vi "main bascula.vi"() -> ()   [LabVIEW 2019]
uses:
  Controls/semafor.ctl
  Controls/Estats.ctl
panel:
  out "Semafor":T1
  out "pedestrian":bool
  in  "Boolean":bool
  in  "stop":bool
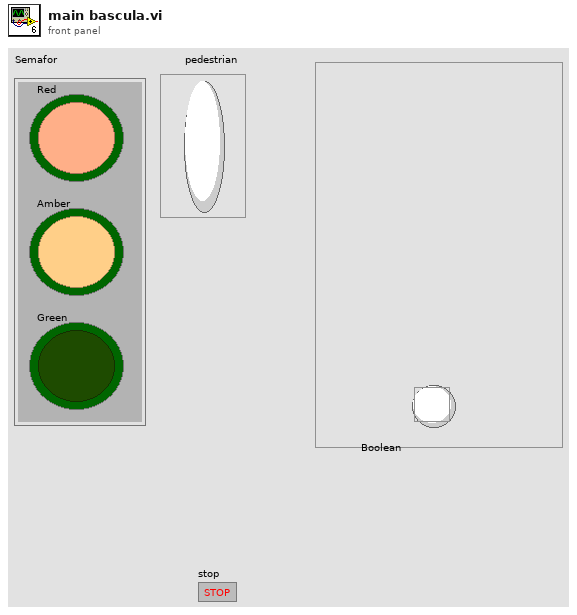
[diagram p1: front panel]
types:
  T1 = typedef "semafor.ctl" = cluster{"Red":bool, "Amber":bool, "Green":bool}
  T2 = typedef "Estats.ctl" = enum16{"Init", "Green", "Amber-red", "red", "amber"}
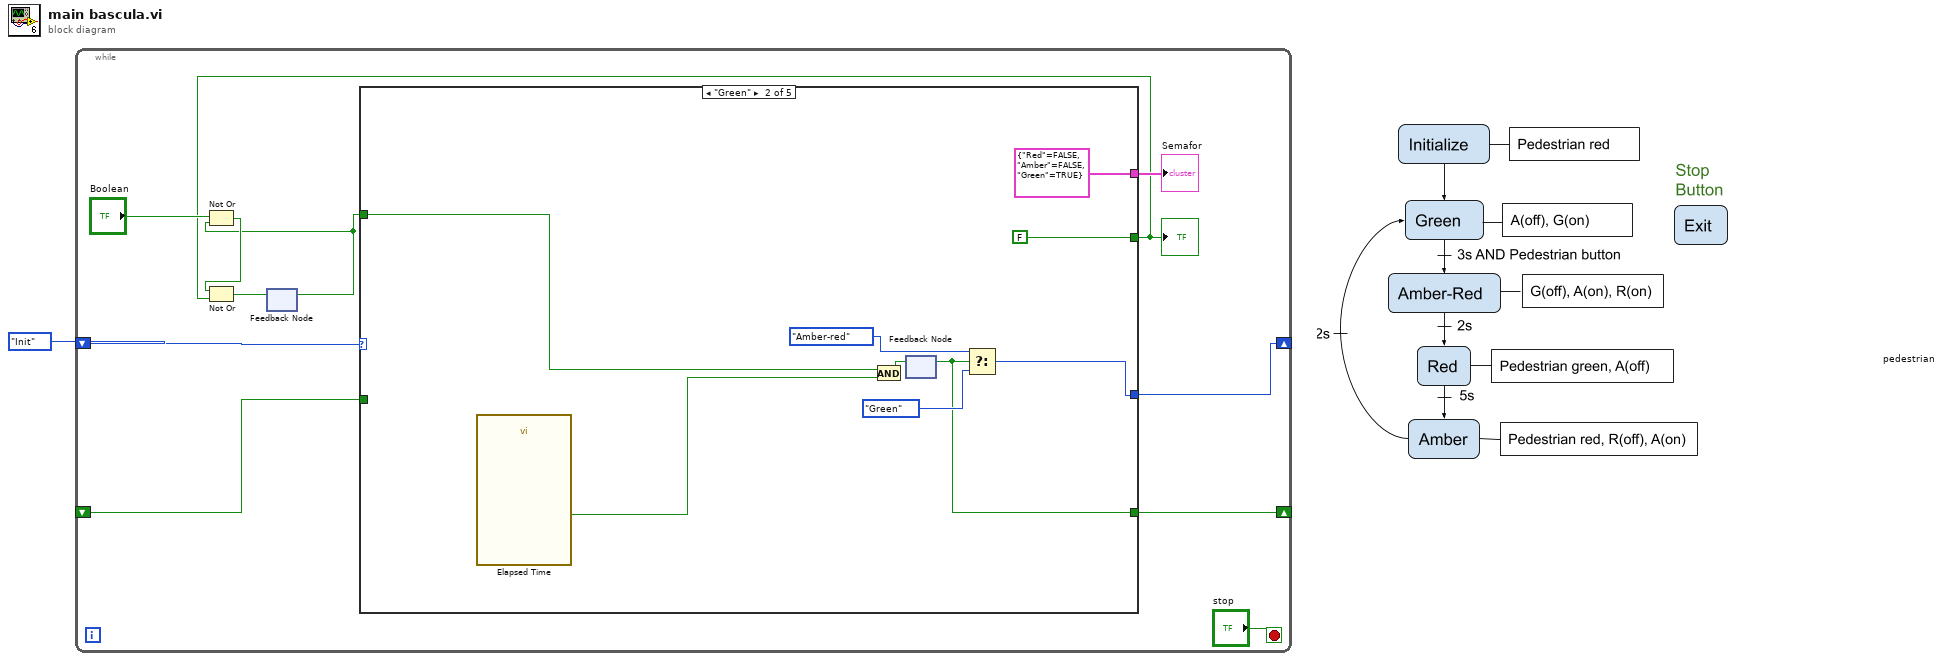
[diagram p0: block diagram]
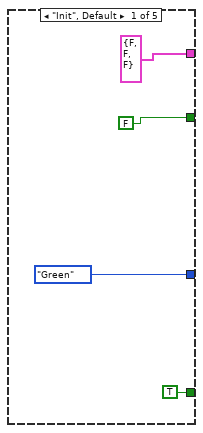
[diagram p2: hidden frame]
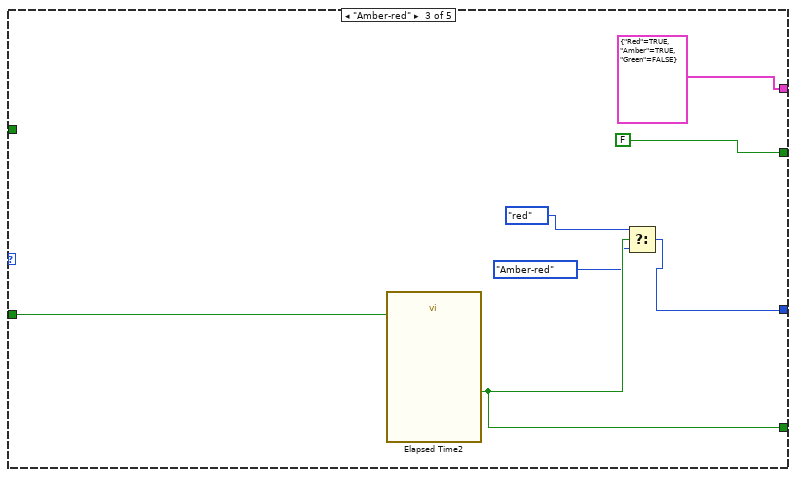
[diagram p3: hidden frame]
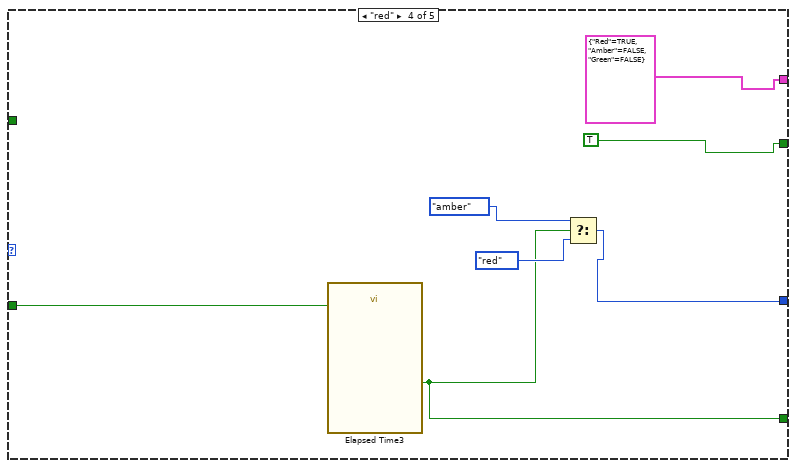
[diagram p4: hidden frame]
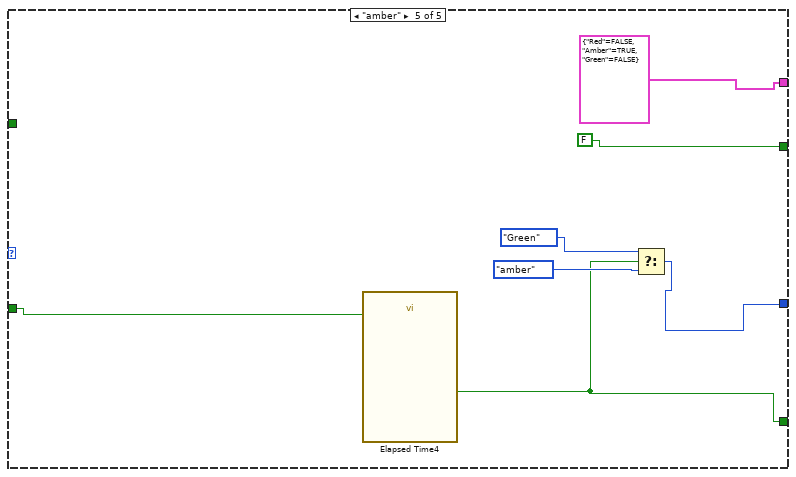
[diagram p5: hidden frame]
diagram:
  n1 = while {
    shift-right: [w11] -> _
    shift-left: _ -> [w10]
    shift-right: [w7] -> _
    shift-left: Estats."Init" ("Enum") -> [w8]
    stop <- "stop" stop-if-true
    n2 = feedback #1() -> (w3:bool)  [unwired: 1 in]
    n3 = Not Or(1:w3, 2:"Boolean") -> (0:w6:bool)
    n4 = case shown="\"Green\"" w8 {
      tunnel: [Estats."Green" ("Enum") w22 w32 w37 w44] -> w7
      tunnel: [TRUE ("Time has Elapsed") w18 w30 w36 w43] -> w11
      tunnel: w10 -> [_ _ w28 w35 w42]
      tunnel: [T1 {"Red"=FALSE, "Amber"=FALSE, "Green"=FALSE} ("Semafor") T1 {"Red"=FALSE, "Amber"=FALSE, "Green"=TRUE} ("Semafor") T1 {"Red"=TRUE, "Amber"=TRUE, "Green"=FALSE} ("Semafor") T1 {"Red"=TRUE, "Amber"=FALSE, "Green"=FALSE} ("Semafor") T1 {"Red"=FALSE, "Amber"=TRUE, "Green"=FALSE} ("Semafor")] -> w9
      tunnel: [FALSE ("pedestrian") FALSE ("pedestrian") FALSE ("pedestrian") TRUE ("pedestrian") FALSE ("pedestrian")] -> w2
      tunnel: w3 -> [_ w17 _ _ _]
      frame "Init", Default {
      }
      frame "Green" {
        n5 = call "Elapsed Time"() -> ("Time has Elapsed"=w23:bool)  [unwired: 12 in, 7 out]
        n6 = And(x=w17, y=w23) -> (x .and. y?=w19:bool)
        n7 = feedback-in #2(w19) -> ()
        n8 = feedback #2() -> (w18:bool)  [unwired: 1 in]
        n9 = Select(t=Estats."Amber-red" ("Enum"), s=w18, f=Estats."Green" ("Enum")) -> (s? t:f=w22:T2)
      }
      frame "Amber-red" {
        n10 = call "Elapsed Time2"("Reset"=w28) -> ("Time has Elapsed"=w30:bool)  [unwired: 11 in, 7 out]
        n11 = Select(t=Estats."red" ("Enum"), s=w30, f=Estats."Amber-red" ("Enum")) -> (s? t:f=w32:T2)
      }
      frame "red" {
        n12 = call "Elapsed Time3"("Reset"=w35) -> ("Time has Elapsed"=w36:bool)  [unwired: 11 in, 7 out]
        n13 = Select(t=Estats."amber" ("Enum"), s=w36, f=Estats."red" ("Enum")) -> (s? t:f=w37:T2)
      }
      frame "amber" {
        n14 = call "Elapsed Time4"("Reset"=w42) -> ("Time has Elapsed"=w43:bool)  [unwired: 11 in, 7 out]
        n15 = Select(t=Estats."Green" ("Enum"), s=w43, f=Estats."amber" ("Enum")) -> (s? t:f=w44:T2)
      }
    }
    "Semafor" <- w9
    "pedestrian" <- w2
    n16 = Not Or(1:w2, 2:w6) -> (0:w4:bool)
    n17 = feedback-in #1(w4) -> ()
  }
